vi "Bounce Window_User Accounts.vi"(11 "User Account Table Path":path) -> ()   [LabVIEW 2015]
uses:
  Control_User account_QData.ctl
  Control_User Accounts_Queue Action.ctl
  <vilib>/Utility/miscctls.llb/LVPointTypeDef.ctl
panel:
  in  "群組：":T1
  out "Queue Data":T2
  in  "User Accounts Table":i32(listbox)=-1
  in  "離開":bool
  in  "修改":bool
  in  "重置密碼":bool
  in  "刪除帳號":bool
  in  "新增帳號":bool
  # "帳號管理"
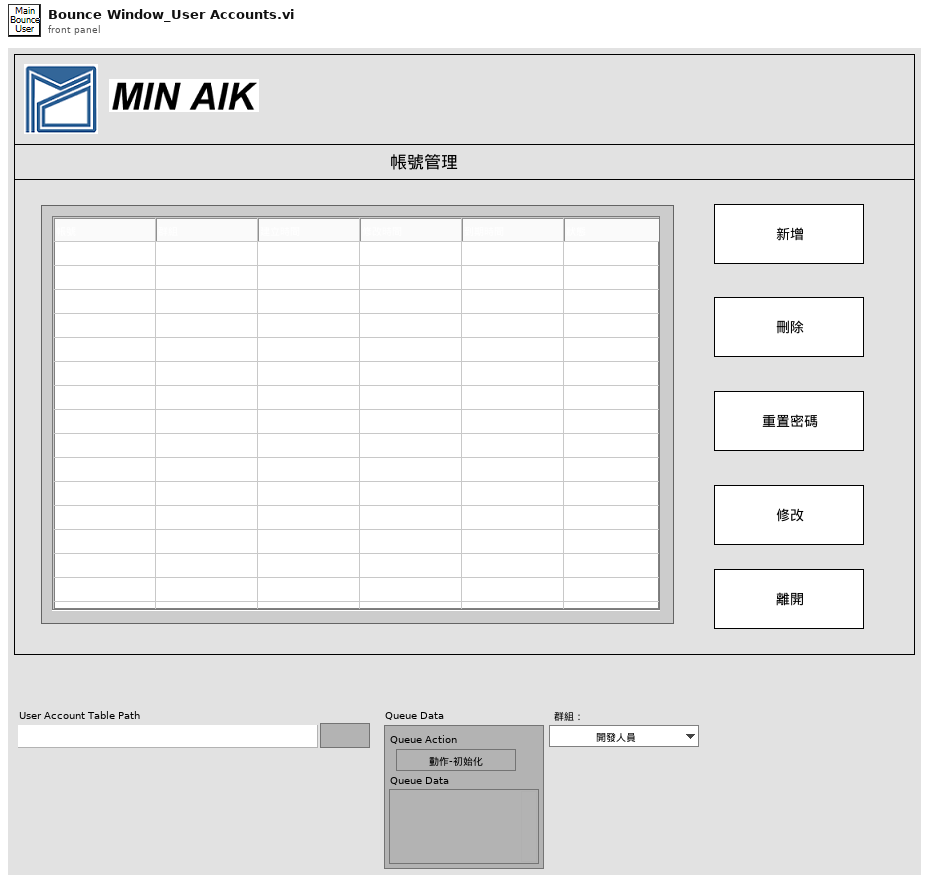
[diagram p1: front panel]
types:
  T1 = typedef "Control_User account_Permissions.ctl" = enum16{"開發人員", "管理者", "工程師", "作業員"}
  T2 = typedef "Control_User account_QData.ctl" = cluster{"Queue Action":T3, "Queue Data":variant}
  T3 = typedef "Control_User Accounts_Queue Action.ctl" = enum16{"動作-初始化", "動作-新增帳號", "動作-刪除帳號", "動作-重置密碼", "動作-修改帳號", "動作-離開", "1.0 檔案", "    1.1 檔案-讀取檔案", "    1.2 檔案-存入檔案", "2.0 Table", "    2.1 Table-初始化", "    2.2 Table-寫入", "    2.3 Table-修改", "    2.4 Table-刪除", "    2.5 Table-結束", "3.0 錯誤", "    3.1 錯誤-顯示錯誤", "4.0 等待", "    4.1 等待-等待時間", "5.0 結束", "    5.1 結束-UI結束", "    5.2 結束-Fun結束", "    5.3 程式結束"}
  T4 = typedef "LVPointTypeDef.ctl" = cluster{"Horizontal":i16, "Vertical":i16}
  T5 = typedef "Control_Bounce Window_User Accounts_Data Action" = enum16{"Initialize", "Set Data", "Set Data Array", "Replace Data", "Delete Data", "Get Data", "Get Data Array"}
  T6 = typedef "Control_User account_Data.ctl" = cluster{"帳號 :":string, "權限等級：":T1, "建立時間：":string, "修改時間：":string, "到期時間：":string, "狀態：":T7, "期限：":T8, "密碼：":string}
  T7 = typedef "Control_User Accounts_Status.ctl" = enum16{"可使用", "不可使用"}
  T8 = typedef "Control_User account_Date.ctl" = enum16{"零天", "一天", "七天", "一個月", "一年", "三年"}
  T9 = typedef "Control_Bounce Window_User Accounts_Table Action" = enum16{"Initialize", "Set Data", "Delete Data", "Replace Data", "Close"}
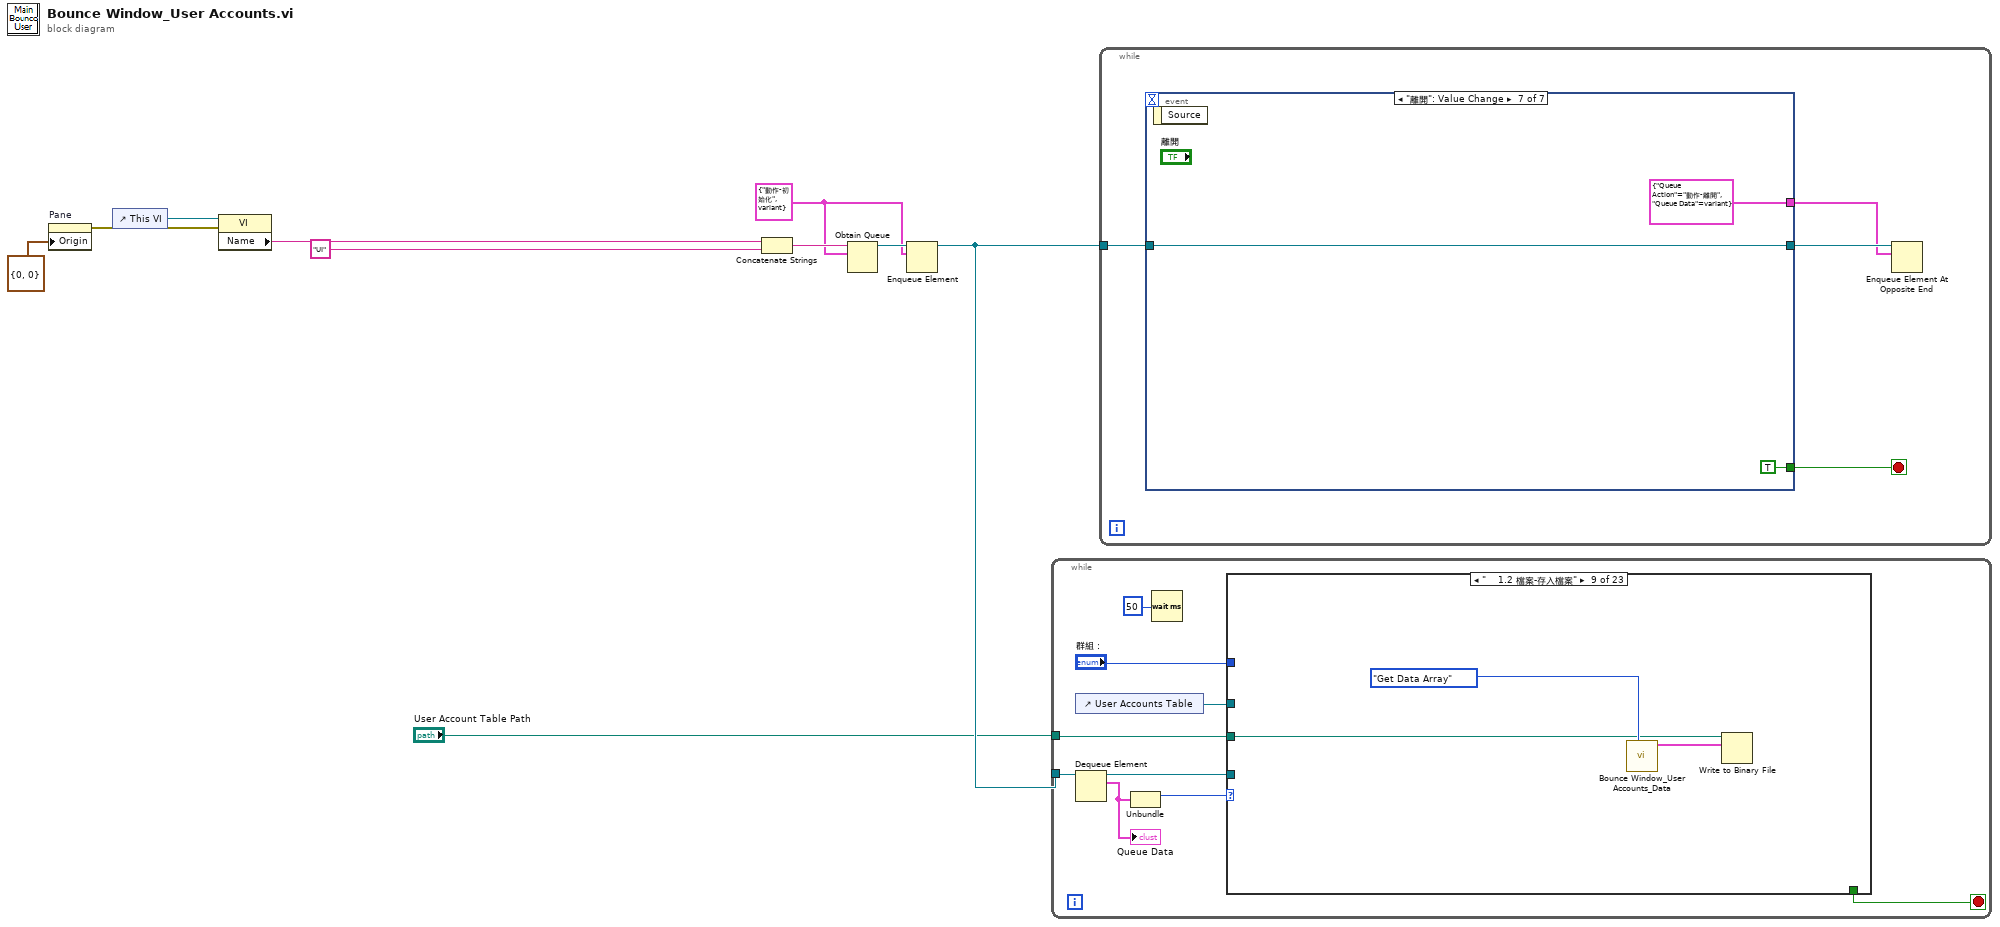
[diagram p0: block diagram]
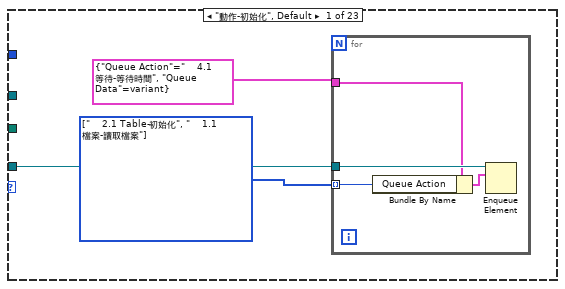
[diagram p2: hidden frame]
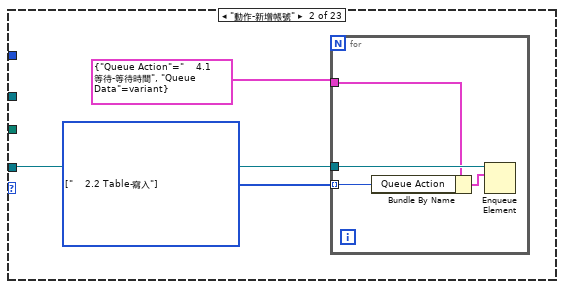
[diagram p3: hidden frame]
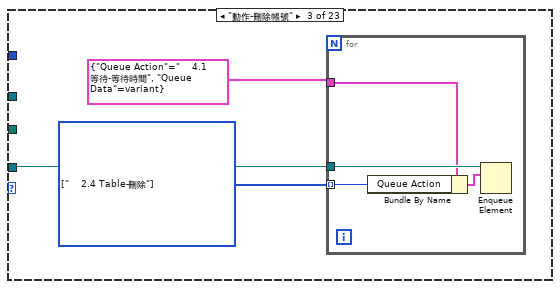
[diagram p4: hidden frame]
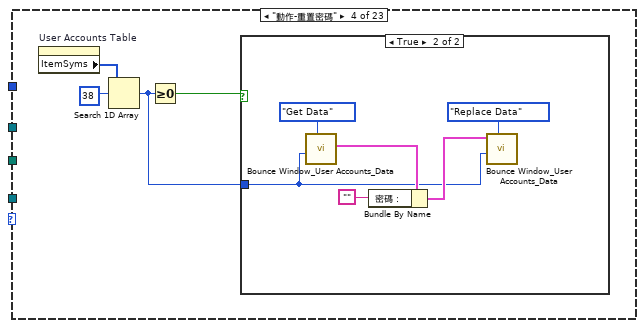
[diagram p5: hidden frame]
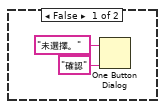
[diagram p6: hidden frame]
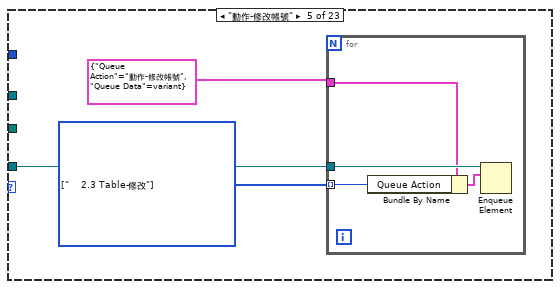
[diagram p7: hidden frame]
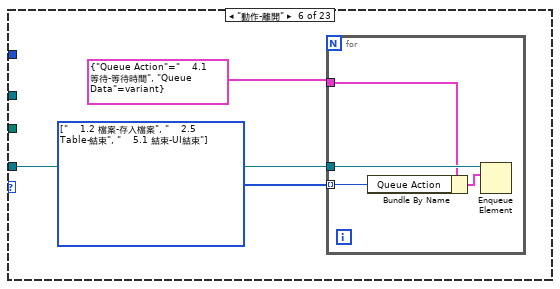
[diagram p8: hidden frame]
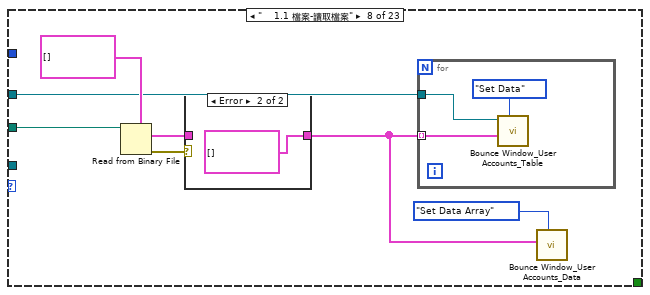
[diagram p10: hidden frame]
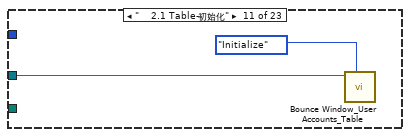
[diagram p13: hidden frame]
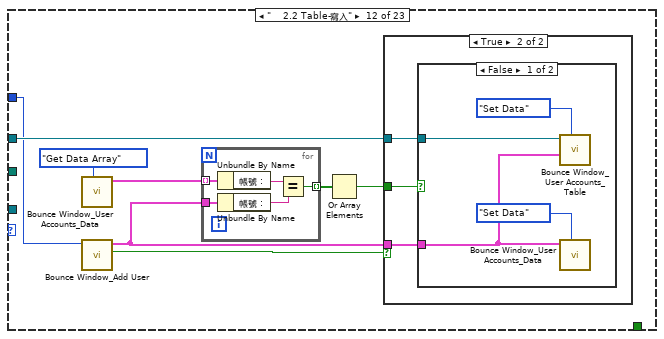
[diagram p14: hidden frame]
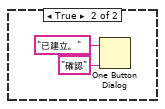
[diagram p16: hidden frame]
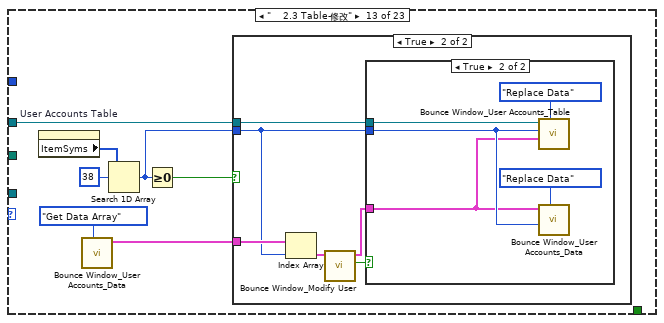
[diagram p17: hidden frame]
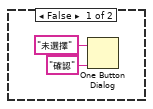
[diagram p18: hidden frame]
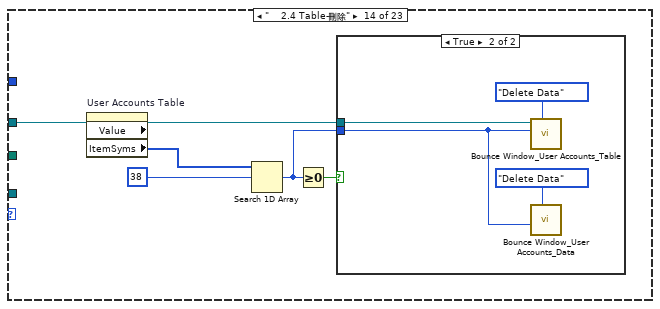
[diagram p20: hidden frame]
diagram:
  w3 = T2 {"Queue Action"=enum."動作-初始化", "Queue Data"=variant} ("Queue Data")
  n1 = property on="Pane" class="Pane"("Origin"=T4 {"Horizontal"=0, "Vertical"=0}) -> (error out=w7:errorcluster)  [unwired: 2 in, 1 out]
  n2 = control-ref of="This VI"() -> (w10:refnum<vi>)
  n3 = property class="VI"(reference=w10, error in=w7) -> ("Name"=w8:string)  [unwired: 2 out]
  n4 = Concatenate Strings(w8, "UI" ("string")) -> (w6:string)
  n5 = Obtain Queue(name (unnamed)=w6, element data type=w3) -> (queue out=w5:refnum<queue>)  [unwired: 3 in, 2 out]
  n6 = Enqueue Element(queue=w5, element=w3) -> (queue out=w4:refnum<queue>)  [unwired: 2 in, 2 out]
  n7 = while {
    tunnel: w4 -> [w18]
    tunnel: "User Account Table Path" -> [w16]
    stop <- w19 stop-if-true
    n8 = control-ref of="User Accounts Table"() -> (w15:refnum<vi>)
    n9 = Dequeue Element(queue=w18) -> (queue out=w17:refnum<queue>, element=w13:T2)  [unwired: 2 in, 2 out]
    "Queue Data" <- w13
    n10 = Unbundle(w13) -> ("Queue Action"=w12:T3)  [unwired: 1 out]
    n11 = Wait (ms)(milliseconds to wait=u32 50) -> ()  [unwired: 1 out]
    n12 = case shown="\"    1.2 檔案-存入檔案\"" w12 {
      tunnel: [_ _ _ _ _ _ _ _ _ _ _ _ _ _ _ _ _ _ _ _ TRUE _ _] -> w19
      tunnel: w17 -> [w20 w27 w35 _ w53 w61 _ _ _ _ _ _ _ _ _ _ _ _ _ _ _ _ _]
      tunnel: w16 -> [_ _ _ _ _ _ _ w73 w79 _ _ _ _ _ _ _ _ _ _ _ _ _ _]
      tunnel: w15 -> [_ _ _ _ _ _ _ w71 _ _ w83 w85 w112 w126 w137 _ _ _ _ _ _ _ _]
      tunnel: "群組：" -> [_ _ _ _ _ _ _ _ _ _ _ w84 _ _ _ _ _ _ _ _ _ _ _]
      frame "動作-初始化", Default {
        w22 = T3[] [enum."    2.1 Table-初始化", enum."    1.1 檔案-讀取檔案"] items=["動作-初始化", "動作-新增帳號", "動作-刪除帳號", "動作-重置密碼", "動作-修改帳號", "動作-離開", "1.0 檔案", "    1.1 檔案-讀取檔案", "    1.2 檔案-存入檔案", "2.0 Table", "    2.1 Table-初始化", "    2.2 Table-寫入", "    2.3 Table-修改", "    2.4 Table-刪除", "    2.5 Table-結束", "3.0 錯誤", "    3.1 錯誤-顯示錯誤", "4.0 等待", "    4.1 等待-等待時間", "5.0 結束", "    5.1 結束-UI結束", "    5.2 結束-Fun結束", "    5.3 程式結束"]
        n13 = for {
          tunnel: w20 -> [w26]
          tunnel: w22 -> [w23] mode=indexing
          tunnel: T2 {"Queue Action"=enum."    4.1 等待-等待時間", "Queue Data"=variant} ("Queue Data") -> [w25]
          n14 = Bundle By Name(cluster=w25, "Queue Action"=w23) -> (w24:T2)
          n15 = Enqueue Element(queue=w26, element=w24) -> ()  [unwired: 2 in, 3 out]
        }
      }
      frame "動作-新增帳號" {
        w29 = T3[] [enum."    2.2 Table-寫入"] items=["動作-初始化", "動作-新增帳號", "動作-刪除帳號", "動作-重置密碼", "動作-修改帳號", "動作-離開", "1.0 檔案", "    1.1 檔案-讀取檔案", "    1.2 檔案-存入檔案", "2.0 Table", "    2.1 Table-初始化", "    2.2 Table-寫入", "    2.3 Table-修改", "    2.4 Table-刪除", "    2.5 Table-結束", "3.0 錯誤", "    3.1 錯誤-顯示錯誤", "4.0 等待", "    4.1 等待-等待時間", "5.0 結束", "    5.1 結束-UI結束", "    5.2 結束-Fun結束", "    5.3 程式結束"]
        n16 = for {
          tunnel: w27 -> [w33]
          tunnel: w29 -> [w30] mode=indexing
          tunnel: T2 {"Queue Action"=enum."    4.1 等待-等待時間", "Queue Data"=variant} ("Queue Data") -> [w32]
          n17 = Bundle By Name(cluster=w32, "Queue Action"=w30) -> (w31:T2)
          n18 = Enqueue Element(queue=w33, element=w31) -> ()  [unwired: 2 in, 3 out]
        }
      }
      frame "動作-刪除帳號" {
        w36 = T3[] [enum."    2.4 Table-刪除"] items=["動作-初始化", "動作-新增帳號", "動作-刪除帳號", "動作-重置密碼", "動作-修改帳號", "動作-離開", "1.0 檔案", "    1.1 檔案-讀取檔案", "    1.2 檔案-存入檔案", "2.0 Table", "    2.1 Table-初始化", "    2.2 Table-寫入", "    2.3 Table-修改", "    2.4 Table-刪除", "    2.5 Table-結束", "3.0 錯誤", "    3.1 錯誤-顯示錯誤", "4.0 等待", "    4.1 等待-等待時間", "5.0 結束", "    5.1 結束-UI結束", "    5.2 結束-Fun結束", "    5.3 程式結束"]
        n19 = for {
          tunnel: w35 -> [w40]
          tunnel: w36 -> [w37] mode=indexing
          tunnel: T2 {"Queue Action"=enum."    4.1 等待-等待時間", "Queue Data"=variant} ("Queue Data") -> [w39]
          n20 = Bundle By Name(cluster=w39, "Queue Action"=w37) -> (w38:T2)
          n21 = Enqueue Element(queue=w40, element=w38) -> ()  [unwired: 2 in, 3 out]
        }
      }
      frame "動作-重置密碼" {
        n22 = property on="User Accounts Table" class="MCListbox (strict)"() -> ("ItemSyms"=w43:i32[])  [unwired: 2 in, 2 out]
        n23 = Search 1D Array(1D array=w43, element=38) -> (index of element=w41:i32)  [unwired: 1 in]
        n24 = Greater Or Equal To 0?(x=w41) -> (x >= 0?=w42:bool)
        n25 = case shown="True" w42 {
          tunnel: w41 -> [_ w47]
          frame False {
            n26 = One Button Dialog(message="未選擇。", button name ("OK")="確認") -> ()  [unwired: 1 out]
          }
          frame True {
            n27 = call "Bounce Window_User Accounts_Data.vi"("Table_Action"=Control_Bounce_Window_User_Accounts_Data_Action."Get Data", "Row"=w47) -> ("User Account Data Out"=w51:T6)  [unwired: 7 in, 2 out]
            n28 = Bundle By Name(cluster=w51, "密碼："="") -> (w48:T6)
            n29 = call "Bounce Window_User Accounts_Data.vi"("Table_Action"=Control_Bounce_Window_User_Accounts_Data_Action."Replace Data", "Row"=w47, "User Account Data In"=w48) -> ()  [unwired: 6 in, 3 out]
          }
        }
      }
      frame "動作-修改帳號" {
        w55 = T3[] [enum."    2.3 Table-修改"] items=["動作-初始化", "動作-新增帳號", "動作-刪除帳號", "動作-重置密碼", "動作-修改帳號", "動作-離開", "1.0 檔案", "    1.1 檔案-讀取檔案", "    1.2 檔案-存入檔案", "2.0 Table", "    2.1 Table-初始化", "    2.2 Table-寫入", "    2.3 Table-修改", "    2.4 Table-刪除", "    2.5 Table-結束", "3.0 錯誤", "    3.1 錯誤-顯示錯誤", "4.0 等待", "    4.1 等待-等待時間", "5.0 結束", "    5.1 結束-UI結束", "    5.2 結束-Fun結束", "    5.3 程式結束"]
        n30 = for {
          tunnel: w53 -> [w59]
          tunnel: w55 -> [w56] mode=indexing
          tunnel: T2 {"Queue Action"=enum."動作-修改帳號", "Queue Data"=variant} ("Queue Data") -> [w58]
          n31 = Bundle By Name(cluster=w58, "Queue Action"=w56) -> (w57:T2)
          n32 = Enqueue Element(queue=w59, element=w57) -> ()  [unwired: 2 in, 3 out]
        }
      }
      frame "動作-離開" {
        w60 = T3[] [enum."    1.2 檔案-存入檔案", enum."    2.5 Table-結束", enum."    5.1 結束-UI結束"] items=["動作-初始化", "動作-新增帳號", "動作-刪除帳號", "動作-重置密碼", "動作-修改帳號", "動作-離開", "1.0 檔案", "    1.1 檔案-讀取檔案", "    1.2 檔案-存入檔案", "2.0 Table", "    2.1 Table-初始化", "    2.2 Table-寫入", "    2.3 Table-修改", "    2.4 Table-刪除", "    2.5 Table-結束", "3.0 錯誤", "    3.1 錯誤-顯示錯誤", "4.0 等待", "    4.1 等待-等待時間", "5.0 結束", "    5.1 結束-UI結束", "    5.2 結束-Fun結束", "    5.3 程式結束"]
        n33 = for {
          tunnel: w61 -> [w66]
          tunnel: w60 -> [w63] mode=indexing
          tunnel: T2 {"Queue Action"=enum."    4.1 等待-等待時間", "Queue Data"=variant} ("Queue Data") -> [w65]
          n34 = Bundle By Name(cluster=w65, "Queue Action"=w63) -> (w64:T2)
          n35 = Enqueue Element(queue=w66, element=w64) -> ()  [unwired: 2 in, 3 out]
        }
      }
      frame "1.0 檔案" {
      }
      frame "    1.1 檔案-讀取檔案" {
        n36 = Read from Binary File(5:T6[] [], 11:w73) -> (0:w69:errorcluster, 2:w68:T6[])  [unwired: 4 in, 2 out]
        n37 = case shown="Error" w69 {
          tunnel: w68 -> [w74 _]
          tunnel: [w74 T6[] []] -> w67
          frame No Error {
          }
          frame Error {
          }
        }
        n38 = for {
          tunnel: w67 -> [w78] mode=indexing
          tunnel: w71 -> [w77]
          n39 = call "Bounce Window_User Accounts_Table.vi"("User Accounts_Action"=Control_Bounce_Window_User_Accounts_Table_Action."Set Data", "User Account Data"=w78, "User Accounts Table"=w77) -> ()  [unwired: 9 in]
        }
        n40 = call "Bounce Window_User Accounts_Data.vi"("Table_Action"=Control_Bounce_Window_User_Accounts_Data_Action."Set Data Array", "Data Array In"=w67) -> ()  [unwired: 7 in, 3 out]
      }
      frame "    1.2 檔案-存入檔案" {
        n41 = call "Bounce Window_User Accounts_Data.vi"("Table_Action"=Control_Bounce_Window_User_Accounts_Data_Action."Get Data Array") -> ("Data Array Out"=w81:T6[])  [unwired: 8 in, 2 out]
        n42 = Write to Binary File(file (use dialog)=w79, data=w81) -> ()  [unwired: 4 in, 3 out]
      }
      frame "2.0 Table" {
      }
      frame "    2.1 Table-初始化" {
        n43 = call "Bounce Window_User Accounts_Table.vi"("User Accounts_Action"=Control_Bounce_Window_User_Accounts_Table_Action."Initialize", "User Accounts Table"=w83) -> ()  [unwired: 10 in]
      }
      frame "    2.2 Table-寫入" {
        n44 = call "Bounce Window_User Accounts_Data.vi"("Table_Action"=Control_Bounce_Window_User_Accounts_Data_Action."Get Data Array") -> ("Data Array Out"=w89:T6[])  [unwired: 8 in, 2 out]
        n45 = call "Bounce Window_Add User.vi"("群組："=w84) -> ("是否新增"=w91:bool, "User Account Data"=w88:T6)  [unwired: 9 in]
        n46 = for {
          tunnel: w89 -> [w96] mode=indexing
          tunnel: w88 -> [w95]
          tunnel: [w92] -> w87 mode=indexing
          n47 = Unbundle By Name(w96) -> ("帳號 :"=w93:string)
          n48 = Unbundle By Name(w95) -> ("帳號 :"=w94:string)
          n49 = Equal?(x=w93, y=w94) -> (x = y?=w92:bool)
        }
        n50 = Or Array Elements(Boolean array=w87) -> (logical OR=w86:bool)
        n51 = case shown="True" w91 {
          tunnel: w85 -> [_ w99]
          tunnel: w88 -> [_ w98]
          tunnel: w86 -> [_ w97]
          frame False {
          }
          frame True {
            n52 = case shown="False" w97 {
              tunnel: w99 -> [w103 _]
              tunnel: w98 -> [w100 _]
              frame False {
                n53 = call "Bounce Window_User Accounts_Table.vi"("User Accounts_Action"=Control_Bounce_Window_User_Accounts_Table_Action."Set Data", "User Account Data"=w100, "User Accounts Table"=w103) -> ()  [unwired: 9 in]
                n54 = call "Bounce Window_User Accounts_Data.vi"("Table_Action"=Control_Bounce_Window_User_Accounts_Data_Action."Set Data", "User Account Data In"=w100) -> ()  [unwired: 7 in, 3 out]
              }
              frame True {
                n55 = One Button Dialog(message="已建立。", button name ("OK")="確認") -> ()  [unwired: 1 out]
              }
            }
          }
        }
      }
      frame "    2.3 Table-修改" {
        n56 = property on="User Accounts Table" class="MCListbox (strict)"() -> ("ItemSyms"=w109:i32[])  [unwired: 2 in, 2 out]
        n57 = call "Bounce Window_User Accounts_Data.vi"("Table_Action"=Control_Bounce_Window_User_Accounts_Data_Action."Get Data Array") -> ("Data Array Out"=w107:T6[])  [unwired: 8 in, 2 out]
        n58 = Search 1D Array(1D array=w109, element=38) -> (index of element=w106:i32)  [unwired: 1 in]
        n59 = Greater Or Equal To 0?(x=w106) -> (x >= 0?=w111:bool)
        n60 = case shown="True" w111 {
          tunnel: w106 -> [_ w115]
          tunnel: w112 -> [_ w120]
          tunnel: w107 -> [_ w119]
          frame False {
            n61 = One Button Dialog(message="未選擇", button name ("OK")="確認") -> ()  [unwired: 1 out]
          }
          frame True {
            n62 = Index Array(array=w119, index=w115) -> (element=w118:T6)
            n63 = call "Bounce Window_Modify User.vi"("User Account Data In"=w118) -> ("是否新增"=w117:bool, "User Account Data"=w116:T6)  [unwired: 9 in]
            n64 = case shown="True" w117 {
              tunnel: w120 -> [_ w125]
              tunnel: w115 -> [_ w122]
              tunnel: w116 -> [_ w121]
              frame False {
              }
              frame True {
                n65 = call "Bounce Window_User Accounts_Table.vi"("User Accounts_Action"=Control_Bounce_Window_User_Accounts_Table_Action."Replace Data", "User Account Data"=w121, "Row"=w122, "User Accounts Table"=w125) -> ()  [unwired: 8 in]
                n66 = call "Bounce Window_User Accounts_Data.vi"("Table_Action"=Control_Bounce_Window_User_Accounts_Data_Action."Replace Data", "Row"=w122, "User Account Data In"=w121) -> ()  [unwired: 6 in, 3 out]
              }
            }
          }
        }
      }
      frame "    2.4 Table-刪除" {
        n67 = property on="User Accounts Table" class="MCListbox (strict)" props=["Value", "ItemSyms"]() -> ("ItemSyms"=w127:i32[])  [unwired: 2 in, 3 out]
        n68 = Search 1D Array(1D array=w127, element=38) -> (index of element=w128:i32)  [unwired: 1 in]
        n69 = Greater Or Equal To 0?(x=w128) -> (x >= 0?=w130:bool)
        n70 = case shown="True" w130 {
          tunnel: w128 -> [_ w136]
          tunnel: w126 -> [_ w135]
          frame False {
            n71 = One Button Dialog(message="未選擇", button name ("OK")="確認") -> ()  [unwired: 1 out]
          }
          frame True {
            n72 = call "Bounce Window_User Accounts_Table.vi"("User Accounts_Action"=Control_Bounce_Window_User_Accounts_Table_Action."Delete Data", "Row"=w136, "User Accounts Table"=w135) -> ()  [unwired: 9 in]
            n73 = call "Bounce Window_User Accounts_Data.vi"("Table_Action"=Control_Bounce_Window_User_Accounts_Data_Action."Delete Data", "Row"=w136) -> ()  [unwired: 7 in, 3 out]
          }
        }
      }
      frame "    2.5 Table-結束" {
        n74 = call "Bounce Window_User Accounts_Table.vi"("User Accounts_Action"=Control_Bounce_Window_User_Accounts_Table_Action."Initialize", "User Accounts Table"=w137) -> ()  [unwired: 10 in]
      }
      frame "3.0 錯誤" {
      }
      frame "    3.1 錯誤-顯示錯誤" {
      }
      frame "4.0 等待" {
      }
      frame "    4.1 等待-等待時間" {
      }
      frame "5.0 結束" {
      }
      frame "    5.1 結束-UI結束" {
      }
      frame "    5.2 結束-Fun結束" {
      }
      frame "    5.3 程式結束" {
      }
    }
  }
  n75 = while {
    tunnel: w4 -> [w143]
    stop <- w142 stop-if-true
    n76 = event shown="[6] \"離開\": Value Change" {
      selector: _ -> [_ _ _ _ _ _ _]
      dyn-events: _ -> [_ _ _ _ _ _ _]
      timeout: _ -> [_ _ _ _ _ _ _]
      tunnel: w143 -> [w144 w159 w161 w163 w165 w167 w169]
      tunnel: [w144 w159 w161 w163 w165 w167 w169] -> w141
      tunnel: [_ _ _ _ _ _ TRUE] -> w142
      tunnel: [_ T2 {"Queue Action"=enum."    4.1 等待-等待時間", "Queue Data"=variant} ("Queue Data") T2 {"Queue Action"=enum."動作-新增帳號", "Queue Data"=variant} ("Queue Data") T2 {"Queue Action"=enum."動作-刪除帳號", "Queue Data"=variant} ("Queue Data") T2 {"Queue Action"=enum."動作-重置密碼", "Queue Data"=variant} ("Queue Data") T2 {"Queue Action"=enum."動作-修改帳號", "Queue Data"=variant} ("Queue Data") T2 {"Queue Action"=enum."動作-離開", "Queue Data"=variant} ("Queue Data")] -> w140
      event Timeout {
        n77 = event-data() -> ()  [unwired: 1 in, 1 out]
      }
      event "User Accounts Table": Mouse Down {
        w151 = 37 ("y")
        n78 = event-data() -> ()  [unwired: 1 in, 1 out]
        n79 = property on="User Accounts Table" class="MCListbox (strict)"() -> ("ItemSyms"=w154:i32[], "Value"=w149:i32)  [unwired: 2 in, 2 out]
        n80 = Index Array(array=w154, index=w149) -> (element=w155:i32)
        n81 = Equal?(x=w155, y=w151) -> (x = y?=w148:bool)
        n82 = Select(t=38 ("y"), s=w148, f=w151) -> (s? t:f=w157:i32)
        n83 = Select(t=u32 16711680 ("Color Box"), s=w148, f=u32 16777225 ("Color Box")) -> (s? t:f=w145:u32)
        n84 = Array Size(array=w154) -> (size(s)=w153:i32)
        n85 = Initialize Array(w151, w153) -> (w152:i32[])
        n86 = Replace Array Subset(array=w152, new element=w157, index=w149) -> (w158:i32[])
        n87 = property on="User Accounts Table" class="MCListbox (strict)"("ItemSyms"=w158, "SelColor"=w145) -> ()  [unwired: 2 in, 2 out]
      }
      event "新增帳號": Value Change {
        n88 = event-data() -> ()  [unwired: 1 in, 1 out]
      }
      event "刪除帳號": Value Change {
        n89 = event-data() -> ()  [unwired: 1 in, 1 out]
      }
      event "重置密碼": Value Change {
        n90 = event-data() -> ()  [unwired: 1 in, 1 out]
      }
      event "修改": Value Change {
        n91 = event-data() -> ()  [unwired: 1 in, 1 out]
      }
      event "離開": Value Change {
        n92 = event-data() -> ()  [unwired: 1 in, 1 out]
      }
    }
    n93 = Enqueue Element At Opposite End(queue=w141, element=w140) -> ()  [unwired: 2 in, 3 out]
  }
